vi "Process-server-message.vi"(8 "error in (no error)":errorcluster, 9 "Message type":T1, 10 "Message":refnum<class "Message.lvclass">, 11 "ModComm in":T2) -> (0 "error out":errorcluster, 3 "ModComm out":T2)   [LabVIEW 2013, in "SLMServer.lvlib" / "SLMServer.lvclass"]
uses:
  SLMServer.lvclass
  Object-reference.ctl
  SA-SLMAPI/Sources/Message.lvclass
  Server-messages.ctl
  SA-SLMAPI/Sources/Error/Error.lvclass
  SA-SLMAPI/Sources/Error/Error.lvclass/Error.ctl
  SA-SLMAPI/Sources/Start-client/Start-client.lvclass
  SA-SLMAPI/Sources/Start-client/Start-client.lvclass/Start-client.ctl
  SA-SLMAPI/Sources/Get-clients/Get-clients.lvclass
  SA-SLMAPI/Sources/Message.lvclass/Message.ctl
  SA-SLMAPI/Sources/Start-client/Read Module path.vi
  SA-SLMAPI/Sources/Start-client/Read Module type.vi
  SA-SLMAPI/Sources/Read Sender type.vi
  SA-SLMAPI/Sources/Read Sender ID.vi
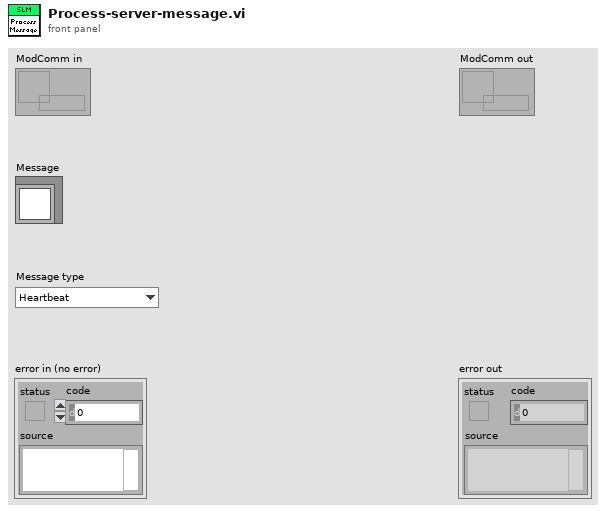
[diagram p1: front panel]
types:
  T1 = typedef "SLMServer.lvlib/SLMServer.lvclass/Server-messages.ctl" = enum16{"Heartbeat", "Error", "Start client", "Client stopped", "Get clients"}
  T2 = typedef "SLMServer.lvlib/SLMServer.lvclass/Object-reference.ctl" = refnum<data-value>
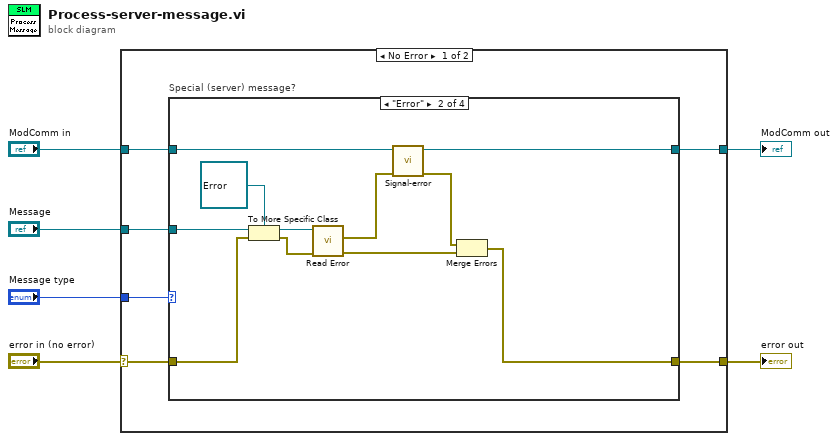
[diagram p0: block diagram]
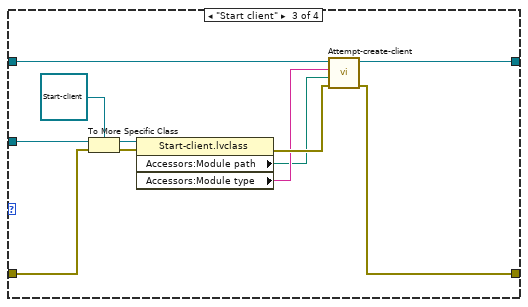
[diagram p3: hidden frame]
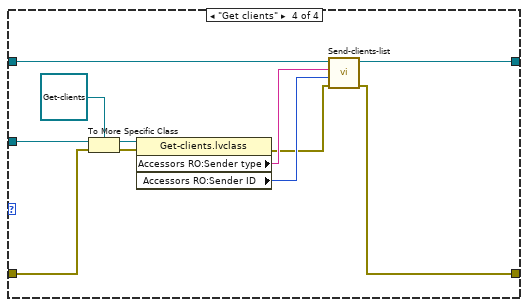
[diagram p4: hidden frame]
diagram:
  n1 = case shown="No Error" "error in (no error)" {
    selector: "error in (no error)" -> [w7 w49]
    tunnel: [w11 w49] -> w5
    tunnel: [w12 w48] -> w3
    tunnel: "ModComm in" -> [w9 w48]
    tunnel: "Message" -> [w8 _]
    tunnel: "Message type" -> [w10 _]
    frame No Error {
      n2 = case "Special (server) message?" shown="\"Error\"" w10 {
        tunnel: [w13 w15 w26 w38] -> w11
        tunnel: [w14 w24 w29 w37] -> w12
        tunnel: w9 -> [w14 w25 w31 w40]
        tunnel: w8 -> [_ w23 w36 w47]
        tunnel: w7 -> [w13 w20 w34 w45]
        frame Default {
        }
        frame "Error" {
          n3 = To More Specific Class(target class=refnum<class "Error.lvclass"> refnum ("Module-communication.lvlib:Error.lvclass"), reference=w23, error in=w20) -> (specific class reference=w21:refnum<class "Error.lvclass">, error out=w19:errorcluster)
          n4 = call "Read Error.vi"("error in (no error)"=w19, "Error in"=w21) -> ("error out"=w16:errorcluster, "Error"=w18:errorcluster)  [unwired: 7 in, 1 out]
          n5 = call "Signal-error.vi"("error in (no error)"=w18, "ModComm in"=w25) -> ("error out"=w17:errorcluster, "ModComm out"=w24:T2)  [unwired: 8 in]
          n6 = Merge Errors(w17, w16) -> (w15:errorcluster)
        }
        frame "Start client" {
          n7 = To More Specific Class(target class=refnum<class "Start-client.lvclass"> refnum ("Module-communication.lvlib:Start-client.lvclass"), reference=w36, error in=w34) -> (specific class reference=w32:refnum<class "Start-client.lvclass">, error out=w33:errorcluster)
          n8 = property class="Start-client.lvclass"(reference=w32, error in=w33) -> (error out=w30:errorcluster, "Accessors:Module path"=w27:path, "Accessors:Module type"=w28:string)  [unwired: 1 out]
          n9 = call "Attempt-create-client.vi"("error in (no error)"=w30, "Module path"=w27, "Module type"=w28, "ModComm in"=w31) -> ("error out"=w26:errorcluster, "ModComm out"=w29:T2)  [unwired: 6 in]
        }
        frame "Get clients" {
          n10 = To More Specific Class(target class=refnum<class "Get-clients.lvclass"> refnum ("Module-communication.lvlib:Get-clients.lvclass"), reference=w47, error in=w45) -> (specific class reference=w43:refnum<class "Get-clients.lvclass">, error out=w44:errorcluster)
          n11 = property class="Get-clients.lvclass"(reference=w43, error in=w44) -> (error out=w39:errorcluster, "Accessors RO:Sender type"=w42:string, "Accessors RO:Sender ID"=w41:i32)  [unwired: 1 out]
          n12 = call "Send-clients-list.vi"("error in (no error)"=w39, "Sender ID"=w41, "Sender"=w42, "ModComm in"=w40) -> ("error out"=w38:errorcluster, "ModComm out"=w37:T2)  [unwired: 6 in]
        }
      }
    }
    frame Error {
    }
  }
  "error out" <- w5
  "ModComm out" <- w3
